vi "Helmholtz2D_FEM_Inpolygon.vi"(8 "yi":dbl, 9 "xi":dbl, 10 "Y":dbl[](array[numeric]), 11 "X":dbl[](array[numeric])) -> (2 "on edge?":bool, 3 "inside?":bool)   [LabVIEW 2017, in "NI_PDE.lvlib"]
uses:
  <vilib>/gmath/NI_PDE.lvlib
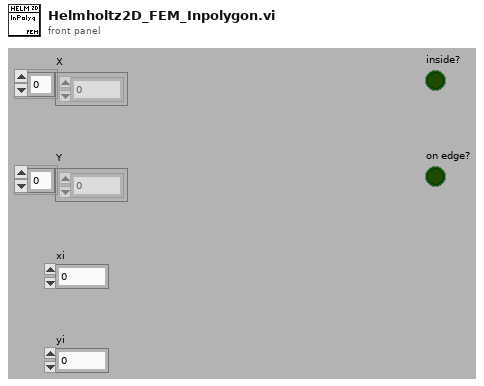
[diagram p1: front panel]
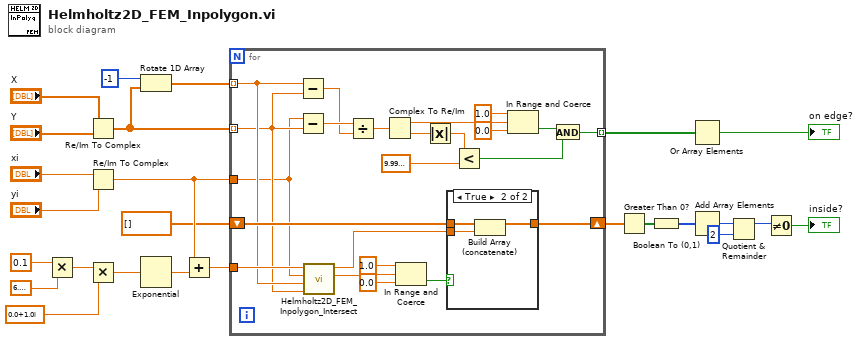
[diagram p0: block diagram]
diagram:
  n1 = Multiply(x=0.1, y=6.283185307179586) -> (x*y=w17:dbl)
  n2 = Re/Im To Complex(1:"Y", 2:"X") -> (0:w24:cdb[])
  n3 = Re/Im To Complex(1:"yi", 2:"xi") -> (0:w22:cdb)
  n4 = Multiply(x=w17, y=cdb 0.0+1.0i) -> (x*y=w19:cdb)
  n5 = Rotate 1D Array(1:w24, 2:-1 ("n")) -> (0:w23:cdb[])
  n6 = Exponential(1:w19) -> (0:w18:cdb)
  n7 = Add(x=w22, y=w18) -> (x+y=w9:cdb)
  n8 = for {
    tunnel: w24 -> [w29] mode=indexing
    tunnel: w23 -> [w30] mode=indexing
    tunnel: w22 -> [w28]
    tunnel: w9 -> [w41]
    shift-right: [w42] -> w2
    shift-left: dbl[] [] -> [w44]
    tunnel: [w27] -> w1 mode=indexing
    n9 = Subtract(x=w30, y=w29) -> (x-y=w39:cdb)
    n10 = Subtract(x=w28, y=w29) -> (x-y=w40:cdb)
    n11 = call <vilib>:"Helmholtz2D_FEM_Inpolygon_Intersect.vi"("x"=w29, "next x"=w30, "p"=w28, "p+dp"=w41) -> ("mu"=w48:dbl, "lambda"=w43:dbl)  [unwired: 6 out]
    n12 = Divide(x=w40, y=w39) -> (x/y=w38:cdb)
    n13 = Complex To Re/Im(x + iy=w38) -> (x=w35:dbl, y=w37:dbl)
    n14 = In Range and Coerce(upper limit=1.0, x=w48, lower limit=0.0) -> (In Range?=w45:bool)  [unwired: 1 out]
    n15 = Absolute Value(x=w37) -> (abs(x)=w36:dbl)
    n16 = case shown="True" w45 {
      tunnel: w44 -> [w49 w52]
      tunnel: w43 -> [_ w51]
      tunnel: [w49 w50] -> w42
      frame False {
      }
      frame True {
        n17 = Build Array (concatenate)(w52, w51) -> (w50:dbl[])
      }
    }
    n18 = Less?(x=w36, y=9.999999717180685e-10) -> (x < y?=w31:bool)
    n19 = In Range and Coerce(upper limit=1.0, x=w35, lower limit=0.0) -> (In Range?=w32:bool)  [unwired: 1 out]
    n20 = And(x=w32, y=w31) -> (x .and. y?=w27:bool)
  }
  n21 = Greater Than 0?(x=w2) -> (x > 0?=w7:bool[])
  n22 = Boolean To (0,1)(Boolean=w7) -> (0, 1=w6:i16[])
  n23 = Or Array Elements(Boolean array=w1) -> (logical OR=→"on edge?":bool)
  n24 = Add Array Elements(numeric array=w6) -> (sum=w5:i16)
  n25 = Quotient & Remainder(x=w5, y=i16 2) -> (x-y*floor(x/y)=w3:i16)  [unwired: 1 out]
  n26 = Not Equal To 0?(x=w3) -> (x != 0?=→"inside?":bool)
